vi "Merge Error.vi"(10 "Error":errorcluster, 11 "TEMPLATE jettl in":refnum<class "TEMPLATE Actor.lvclass">) -> (3 "TEMPLATE jettl out":refnum<class "TEMPLATE Actor.lvclass">)   [LabVIEW 2021, in "_Template.lvlib" / "Templates.lvlib" / "TEMPLATE Actor.lvlib" / "TEMPLATE Actor.lvclass"]
uses:
  TEMPLATE Actor.lvclass
  TEMPLATE Actor.lvclass/TEMPLATE Actor.ctl
  jettl/jettl/jettl/jettl.lvclass
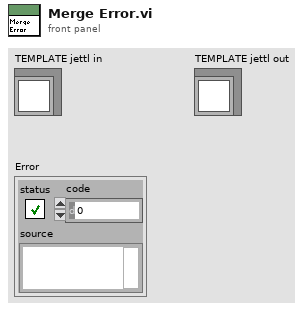
[diagram p1: front panel]
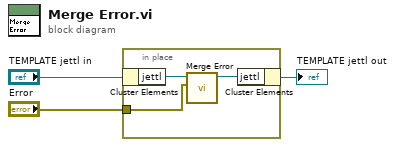
[diagram p0: block diagram]
diagram:
  n1 = in-place {
    in-place-border: "Error" -> [w4]
    n2 = in-place-cluster #1("TEMPLATE jettl in") -> ("jettl"=w6:refnum<class "jettl.lvclass">)
    n3 = call-dynamic "Merge Error.vi"("Error"=w4, "Merge Error in"=w6) -> ("Merge Error out"=w5:refnum<class "jettl.lvclass">)  [unwired: 9 in]
    n4 = in-place-cluster #1("jettl"=w5) -> (→"TEMPLATE jettl out":refnum<class "TEMPLATE Actor.lvclass">)
  }
